vi "Init_CtlLookup.vi"   [LabVIEW 2018, in "CtlReferences.lvlib" / "CtlReferences.lvclass"]
doc: "Polymorphic VI which will generate all of the Control Refs for a give VI\n\nInputs:\n- VI Ref\n- VI Path\n- Nothing [Uses caller VI]"
uses:
  CtlReferences.lvclass
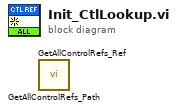
[diagram p0: block diagram]
diagram:
  n1 = call "GetAllControlRefs_Path.vi"() -> ()  [unwired: 10 in, 2 out]
  n2 = call "GetAllControlRefs_Ref.vi"() -> ()  [unwired: 10 in, 2 out]
